vi "tokenScan.vi"() -> ()   [LabVIEW 2021]
panel:
  out "output 1":i32
  out "number 3":i32
  out "result string":string
  out "number 2":i32
  out "number":i32
  out "Out":string
  in  "stop":bool
  in  "Numeric":dbl
  in  "String 3":string
  in  "String 2":string
  in  "String":string
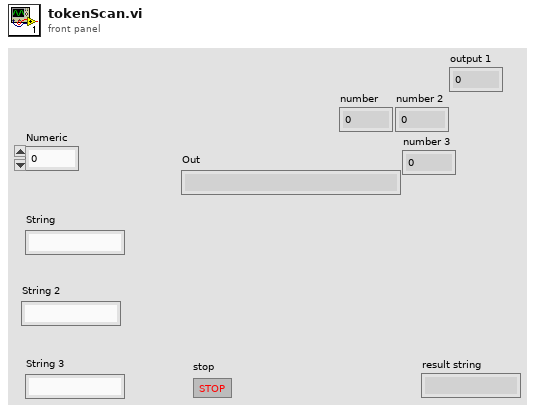
[diagram p1: front panel]
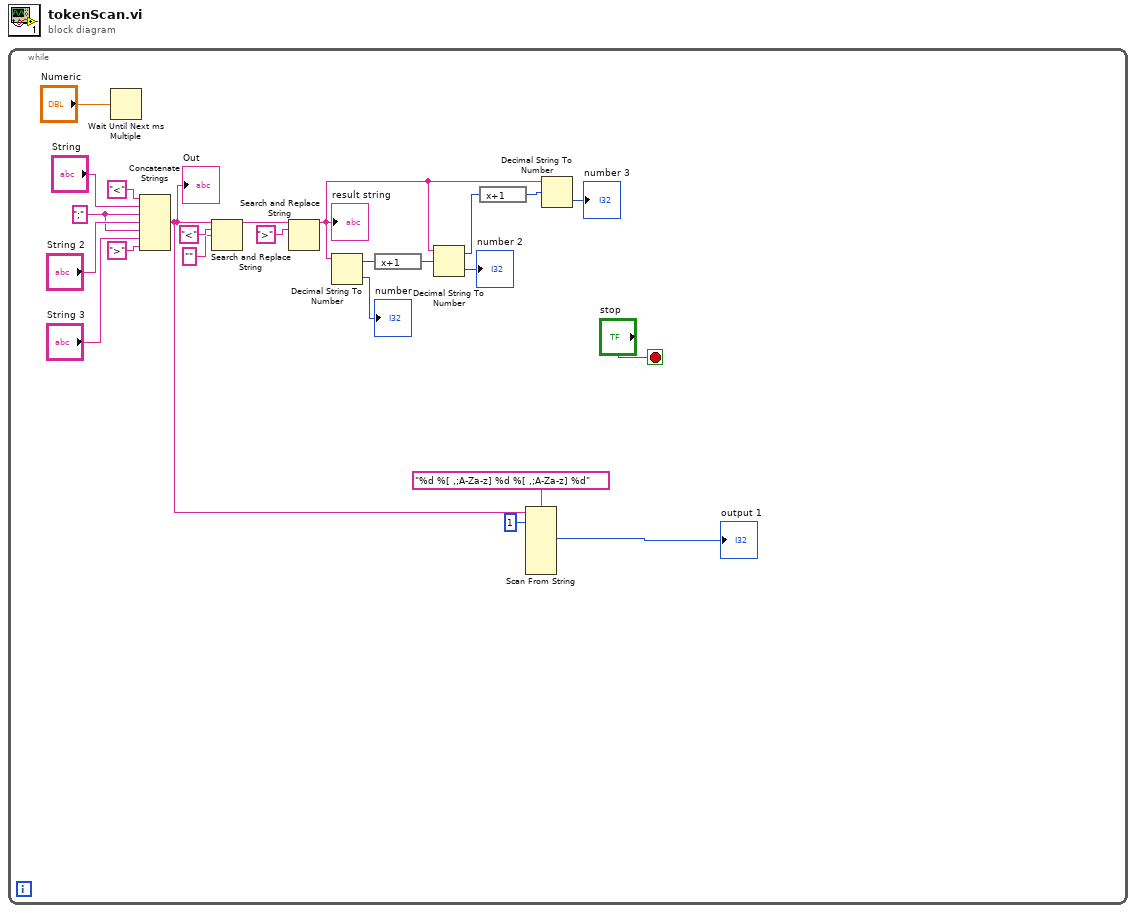
[diagram p0: block diagram]
diagram:
  n1 = while {
    stop <- "stop" stop-if-true
    w17 = ";"
    n2 = Wait Until Next ms Multiple(millisecond multiple="Numeric") -> ()  [unwired: 1 out]
    n3 = Concatenate Strings("<", "String", w17, "String 2", w17, "String 3", ">") -> (w4:string)
    "Out" <- w4
    n4 = Search and Replace String(input string=w4, search string="<", replace string="" ("replace string (\"\")")) -> (result string=w12:string)  [unwired: 5 in, 3 out]
    n5 = Search and Replace String(input string=w12, search string=">") -> (result string=w8:string)  [unwired: 6 in, 3 out]
    "result string" <- w8
    n6 = Decimal String To Number(string=w8) -> (offset past number=w10:i32, number=→"number":i32)  [unwired: 2 in]
    n7 = expression code="x+1"(w10) -> (w9:i32)
    n8 = Decimal String To Number(string=w8, offset=w9) -> (offset past number=w7:i32, number=→"number 2":i32)  [unwired: 1 in]
    n9 = expression code="x+1"(w7) -> (w6:i32)
    n10 = Scan From String(format string="%d %[ ,;A-Za-z] %d %[ ,;A-Za-z] %d", input string=w4, initial scan location=u32 1) -> (output 1=→"output 1":i32)  [unwired: 10 in, 3 out]
    n11 = Decimal String To Number(string=w8, offset=w6) -> (number=→"number 3":i32)  [unwired: 1 in, 1 out]
  }
